vi "Remove Observer.vi"(8 "error in (no error)":errorcluster, 10 "Observer Pattern Actor Interface.lvlib:Observer.lvclass":refnum<class "Observer.lvclass">, 11 "WT1600 in":refnum<class "WT1600.lvclass">) -> (0 "error out":errorcluster, 3 "WT1600 out":refnum<class "WT1600.lvclass">)   [LabVIEW 2012]
uses:
  Observer Pattern Actor Template/Observer/Observer.lvclass
  WT1600.lvclass
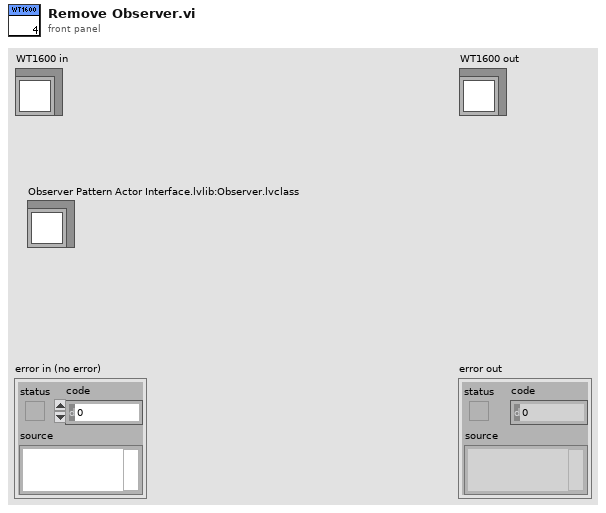
[diagram p1: front panel]
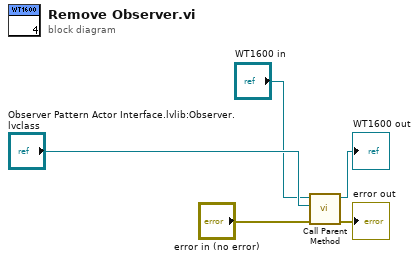
[diagram p0: block diagram]
diagram:
  n1 = call-parent "Call Parent Method"("error in (no error)"="error in (no error)", "Observer Pattern Actor Interface.lvlib:Observer.lvclass"="Observer Pattern Actor Interface.lvlib:Observer.lvclass", "Subject in"="WT1600 in") -> ("error out"=→"error out":errorcluster, "Subject out"=→"WT1600 out":refnum<class "WT1600.lvclass">)  [unwired: 7 in]
